vi "DRAW FP DINERO IN UI.vi"(8 "error in (no error)":errorcluster, 11 "Dinero in":refnum<class "Dinero.lvclass">) -> (0 "error out":errorcluster, 3 "Dinero out":refnum<class "Dinero.lvclass">)   [LabVIEW 2020, in "Dinero.lvlib" / "Dinero.lvclass"]
uses:
  Dinero.lvclass
  Dinero.lvclass/Dinero.ctl
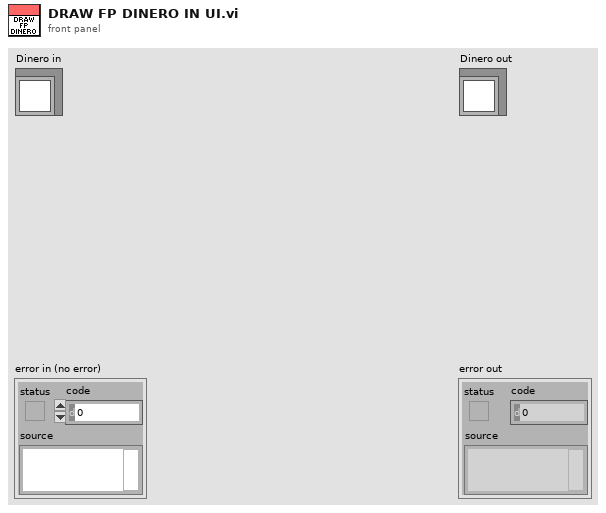
[diagram p1: front panel]
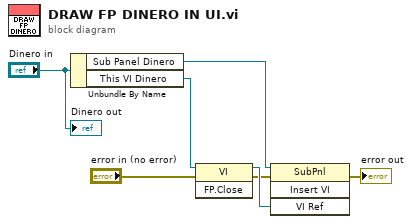
[diagram p0: block diagram]
diagram:
  n1 = Unbundle By Name("Dinero in") -> ("Sub Panel Dinero"=w3:refnum<vi>, "This VI Dinero"=w5:refnum<vi>)
  n2 = invoke class="VI" method="FP.Close"(reference=w5, error in="error in (no error)") -> (reference out=w6:refnum<vi>, error out=w4:errorcluster)  [unwired: 1 in, 1 out]
  n3 = invoke class="SubPnl" method="Insert VI"(reference=w3, error in=w4, "VI Ref"=w6) -> (error out=→"error out":errorcluster)  [unwired: 1 in, 3 out]
  "Dinero out" <- "Dinero in"
